vi "trace_math_spectra_divide.vi"(0 "reference in":refnum<class "OSA.lvclass">, 1 "spectrum 1 dividend trace idx":u32, 2 "spectrum 2 divisor trace idx":u32, 5 "error in (no error)":errorcluster) -> (13 "global dividend trace idx":u32, 14 "reference out":refnum<class "OSA.lvclass">, 19 "error out":errorcluster)   [LabVIEW 2010, in "OSA.lvclass"]
doc: "This divides two spectra On return will spectrum1 be equal to spectrum1 / spectrum2 \n\nParameters\n\nspectrum1: the dividend and also the output spectrum. \n\nspectrum2: the divisor. \n\nReturns FTS_ERROR_DIMENSION_MISMATCH if the lengths of the two spectra are different FTS_ERROR_DIMENSION_MISMATCH if the x-axis values of the two spectra differ FTS_SUCCESS on success"
uses:
  OSA.lvclass
  typeDef/acq_dataType.ctl
  FTSLib.dll
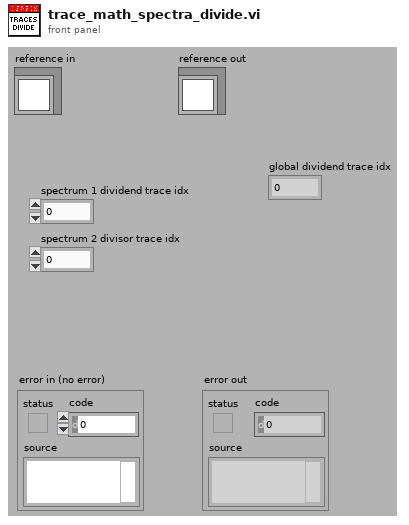
[diagram p1: front panel]
types:
  T1 = typedef "OSA.lvclass/acq_dataType.ctl" = enum16{"none", "interferogram", "spectrum"}
  T2 = typedef "OSA.lvclass/ObjectAttributes.ctl" = cluster{"Stop":bool, "dataType":T1, "spectrometerIdx":u16, "buffer size interferogram":i32, "interferogram":cluster{"new":bool, "plot_x_ min":sgl, "plot_x_max":sgl, "plot_y_min":sgl, "plot_y_max":sgl, "Graph Intrfrgrm":T3, "timeStamp":u32, "signal (%)":dbl, "traces":cluster{"idx":u32, "broadBand":bool, "monoChromatic":bool, "peakToPeakSignal":dbl, "peakToPeakPos":dbl}[], "traces idx last":i32}, "spectrum":cluster{"new":bool, "plot_x_min":sgl, "plot_x_max":sgl, "plot_unit_x":T4, "plot_unit_y":T5, "plot_y_min":sgl, "plot_y_max":sgl, "Graph Spectrum":T3, "timeStamp":u32, "X_VAL_OPTIONS":enum16{"MIN_MAX", "ARRAY"}, "traces":cluster{"idx":u32}[], "traces idx last":i32}, "Thorlabs_OSA_64.lvclass:queue_action.ctlqueue ref":refnum<queue>, "action":T6, "plot zoom step":dbl, "buffer semaphore":T7, "acq stopped":bool, "dataType active":T1, "temperature (degr C)":sgl, "pressure (hPa)":sgl, "rel humidity (%)":sgl, "settings":cluster{"resolution":u16, "sensitivity":u16, "Average":bool, "average nr":u32, "apodisation":T8, "acq delay (ms)":u32, "airMesure":T9, "wmtr on":bool, "intfgrm_smooth_width":u16, "intfgrm_smooth_nrOfPasses":u16, "intfgrm_smooth":T10, "phaseCorrection":T11, "zeroFill":u8, "spectr_smooth":T10, "spectr_smooth_width":u16, "spectr_smooth_nrOfPasses":u16, "resolution (/cm)":sgl, "REF wavelength, (nm)":dbl, "gain_idx":u16, "gainAuto":bool, "gain_relative":dbl, "PD sensitivity mode":T12, "PD senseMode implemented":bool, "SensorTemperature implemented":bool, "SensorPressure implemented":bool, "SensorHumidity implemented":bool, "attenuationAuto":bool, "attenuationOnOff":bool, "attenuationAvailable":bool, "offsetAvailable":bool, "offset":i32, "offset max":u16}, "peaks position":sgl[], "peaks width":sgl[], "peaks height":sgl[], "peaks max nr":u32, "peaks latest nr":i32, "peaks new":bool, "power":dbl, "power new":bool, "path":string, "wavelength (WNr)":dbl, "wavelength new":bool, "buffer size spectrum":i32, "status":string, "VI reference":refnum<vi>, "funcPointer":u64, "libraryPointer":u64, "singleAcquisition":bool, "coherenceLength (cm)":dbl, "coherenceLength new":bool, "spectrometer model":string, "spectrometer serial nr":string, "peaks thld left":sgl[], "peaks thld right":sgl[], "coherenceLength error (cm)":dbl, "ADC bits":u16, "peaks position centroid":sgl[], "peaks height centroid":sgl[], "OSA series":T13, "channel index spectrum":u16, "spectrometer rangeLow, (/cm)":dbl, "spectrometer rangeHigh, (/cm)":dbl, "channel index interferogram":u16}
  T3 = typedef "OSA.lvclass/graph_intensity.ctl" = refnum<vi>
  T4 = typedef "OSA.lvclass/spectrum_x_unit.ctl" = enum16{"wavenr/cm", "THz", "eV", "nm_air", "nm_vac"}
  T5 = typedef "OSA.lvclass/y_unit.ctl" = enum16{"ADC counts", "dBm pwr absolute", "dBm pwr density", "mW pwr absolute", "mW pwr density"}
  T6 = typedef "OSA.lvclass/queue_action.ctl" = enum16{"none", "stop", "GUI_plotInterferogram", "GUI_plotSpectrum", "GUI_plotInterferogramRescale", "GUI_plotSpectrumRescale", "GUI_plotInterferogramReset", "GUI_plotSpectrumReset", "GUI_plotInterferogramAutoScaleY", "GUI_plotSpectrumAutoScaleY", "GUI_plotInterferogramZoomOut", "GUI_plotSpectrumZoomOut", "GUI_plotInterferogramPane", "GUI_plotSpectrumPane", "GUI_plotInterferogramZoomMouse", "GUI_plotSpectrumZoomMouse", "GUI_spectrumChannelType", "GUI_channel", "ENVIRONMENT temperature", "ENVIRONMENT pressure", "MODE_resolution set", "MODE_resolution get", "MODE_sensitivity set", "MODE_sensitivity get", "MODE_PDTemperature set", "MODE_PDTemperature get", "REBOOT/RESET firmware", "ACQASYNC_acquireSingleSpectrum", "ACQASYNC_continuous start", "ACQASYNC_continuous stop\n", "ACQASYNC_get last interferogram", "ACQASYNC_get last spectrum", "ACQASYNC_get last waveNr", "ACQOPT_interferogram smoothing set", "ACQOPT_interferogram smoothing get", "ACQOPT_spectrum smoothing set", "ACQOPT_spectrum smoothing get", "ACQOPT_apodisation type set", "ACQOPT_apodisation type get", "ACQOPT_phase correction type set", "ACQOPT_phase correction type get", "ACQOPT_acqIntervall_set", "ACQOPT_acqIntervall_get", "ACQOPT_average spectrum set", "ACQOPT_average spectrum get", "ACQOPT_rolling average set", "ACQOPT_rolling average get", "ACQOPT_zero fill factor set", "ACQOPT_zero fill factor get", "ACQOPT_cycle counting set", "ACQOPT_cycle counting get", "ACQOPT_air measure option set", "ACQOPT_air measure option get", "ACQOPT_gainLevel auto get", "ACQOPT_gainLevel auto set", "ACQOPT_gainLevel get", "ACQOPT_gainLevel set", "ACQOPT_getAll", "INSTRUMENT_PROPERTY_range_WaveNr_min", "INSTRUMENT_PROPERTY_range_WaveNr_max", "INSTRUMENT_PROPERTY_reference_wavelength_cm^-1", "INSTRUMENT_PROPERTY_samplesPerRefPeriod", "INSTRUMENT_PROPERTY_resolution_waveNrPercm", "INSTRUMENT_PROPERTY_availableGainLevels", "INSTRUMENT_PROPERTY_status", "CONVERT", "ANALYSE_POWER", "ANALYSE_PEAKS", "ANALYSE_WAVELENGTH", "ANALYSE_SPECTRUM", "ANALYSE_INTERFEROGRAM", "ANALYSE_COHERENCE_LENGTH", "MATH", "MATH_power", "MATH_peaks", "FILE", "miscellaneous"}
  T7 = typedef "Semaphore RefNum" = refnum<k1>
  T8 = typedef "OSA.lvclass/apodisation.ctl" = enum16{"NONE", "NORTON_BEER_WEAK", "NORTON_BEER_MEDIUM", "NORTON_BEER_STRONG", "TRIANGULAR", "COSINE", "HANN", "HAMMING", "BLACKMANHARRIS3", "BLACKMANHARRIS4", "GAUSSIAN"}
  T9 = typedef "OSA.lvclass/airMeasure.ctl" = enum16{"TEMPERATURE", "PRESSURE"}
  T10 = typedef "OSA20X_misc.lvlib/interferogram_smoothing.ctl" = enum16{"NONE", "BINOMIAL", "SAVITSKY_GOLAY", "FOURIER", "MOVING_AVERAGE", "GAUSSIAN"}
  T11 = typedef "OSA.lvclass/phaseCorrection.ctl" = enum16{"NONE", "MERTZ", "FORMAN", "MERTZ_FILE", "FORMAN_FILE", "FUTURE COMP."}
  T12 = typedef "OSA20X_misc.lvlib/PDTemperatureMode.ctl" = enum16{"cool: better sensitivity/noise floor", "warm: extended wl range"}
  T13 = typedef "OSA.lvclass/OSA_series.ctl" = enum16{"OSA200", "OSA300", "UNKNOWN"}
  T14 = cluster{"idx":u32, "broadBand":bool, "monoChromatic":bool, "peakToPeakSignal":dbl, "peakToPeakPos":dbl}[]
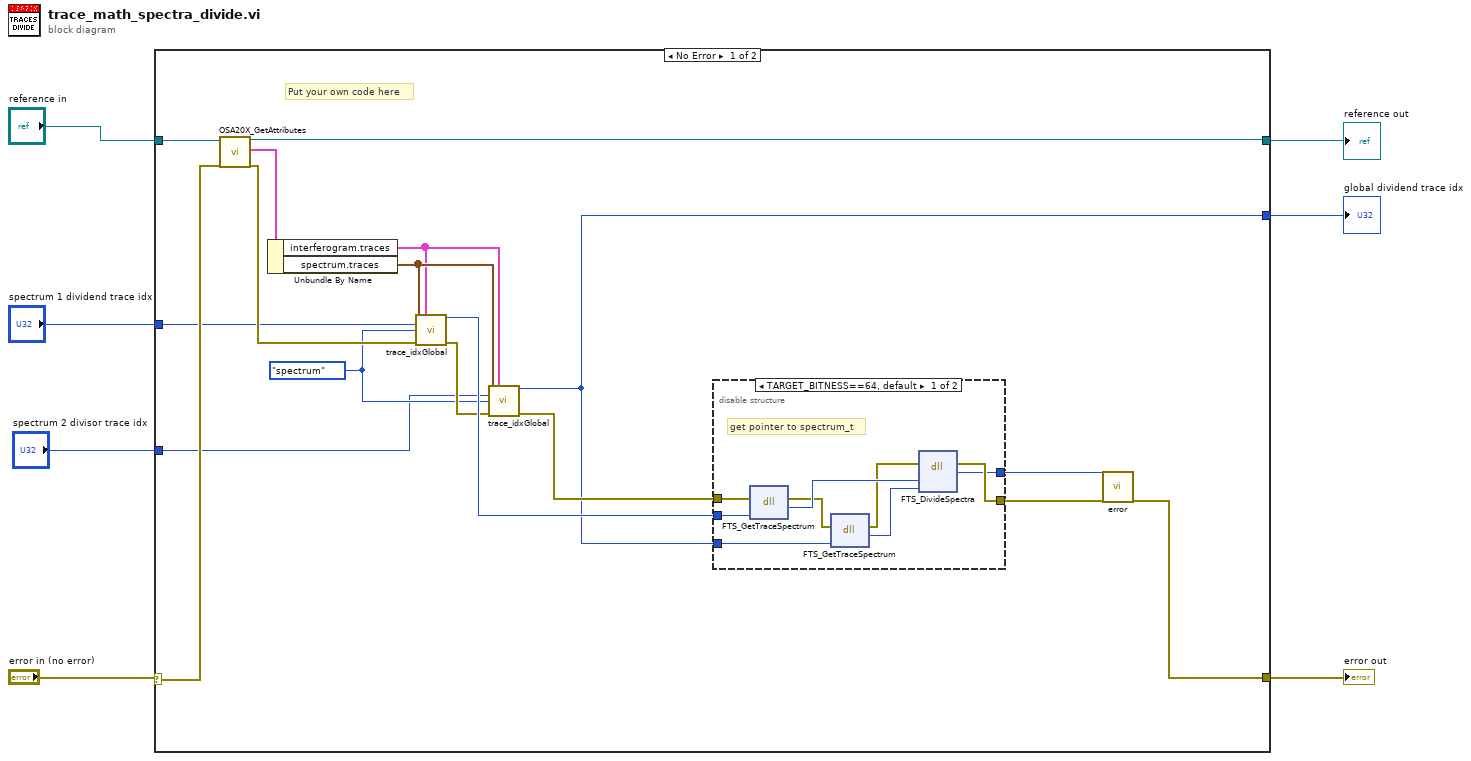
[diagram p0: block diagram]
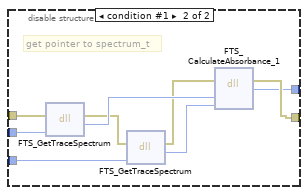
[diagram p2: hidden frame]
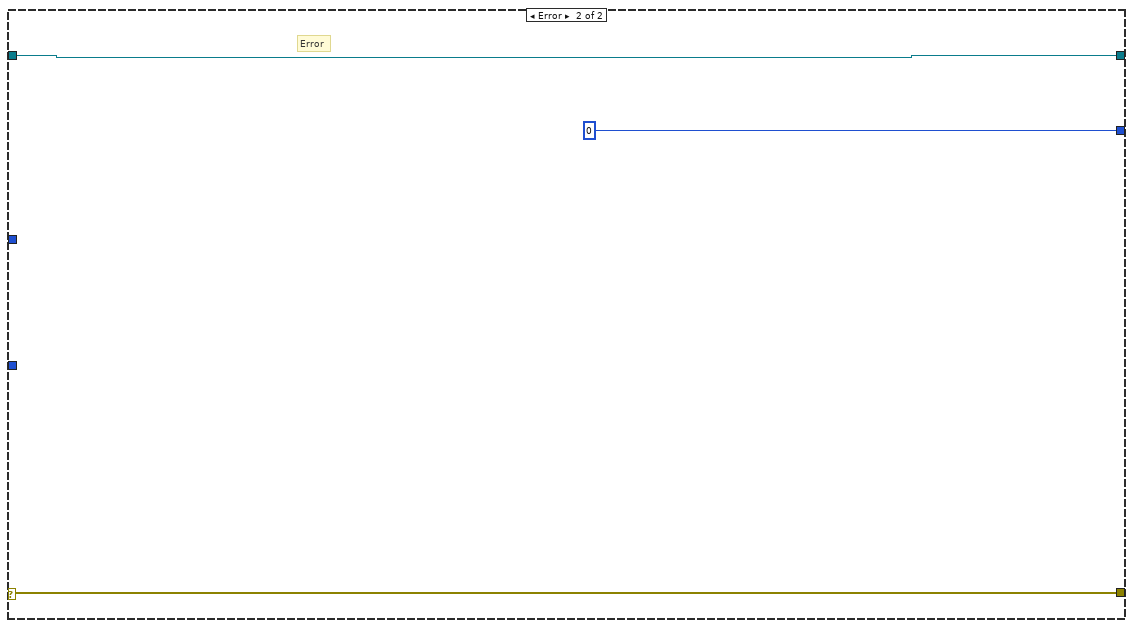
[diagram p3: hidden frame]
diagram:
  n1 = case shown="No Error" "error in (no error)" {
    selector: "error in (no error)" -> [w20 w45]
    tunnel: [w24 w45] -> w7
    tunnel: "reference in" -> [w22 w44]
    tunnel: [w21 w44] -> w2
    tunnel: "spectrum 1 dividend trace idx" -> [w18 _]
    tunnel: [w8 u32 0 ("global trace idx")] -> w3
    tunnel: "spectrum 2 divisor trace idx" -> [w9 _]
    frame No Error {
      w10 = acq_dataType."spectrum" ("dataType")
      # "Put your own code here"
      n2 = call "OSA20X_GetAttributes.vi"("reference in"=w22, "error in (no error)"=w20) -> ("reference out"=w21:refnum<class "OSA.lvclass">, "Data"=w23:T2, "error out"=w19:errorcluster)  [unwired: 14 in, 1 out]
      n3 = Unbundle By Name(w23) -> ("interferogram.traces"=w11:T14, "spectrum.traces"=w12:cluster{"idx":u32}[])
      n4 = call "trace_idxGlobal.vi"("traces_spectrum"=w12, "traces_interferogram"=w11, "trace idx"=w18, "dataType"=w10, "error in (no error)"=w19) -> ("global trace idx"=w15:u32, "error out"=w14:errorcluster)  [unwired: 9 in]
      n5 = call "trace_idxGlobal.vi"("traces_spectrum"=w12, "traces_interferogram"=w11, "trace idx"=w9, "dataType"=w10, "error in (no error)"=w14) -> ("global trace idx"=w8:u32, "error out"=w13:errorcluster)  [unwired: 9 in]
      n6 = disable-structure shown="TARGET_BITNESS==64, default" {
        disable-tunnel: w15 -> [w33 w35]
        disable-tunnel: w13 -> [w31 w36]
        disable-tunnel: [w30 w38] -> w17
        disable-tunnel: [w29 w37] -> w16
        disable-tunnel: w8 -> [w26 w34]
        frame condition #0 (active) {
          # "get pointer to spectrum_t"
          n7 = dll-call lib="FTSLib.dll" fn="FTS_GetTraceSpectrum"(error in=w31, "traceIdx"=w33) -> (error out=w28:errorcluster, "spectrum_t_pointer"=w32:u64)  [unwired: 3 in, 1 out]
          n8 = dll-call lib="FTSLib.dll" fn="FTS_GetTraceSpectrum"(error in=w28, "traceIdx"=w26) -> (error out=w27:errorcluster, "spectrum_t_pointer"=w25:u64)  [unwired: 3 in, 1 out]
          n9 = dll-call lib="FTSLib.dll" fn="FTS_DivideSpectra"(error in=w27, "spectrum_t_pointer"=w32, "spectrum_t_pointer"=w25) -> (error out=w30:errorcluster, "returnVal"=w29:i32)  [unwired: 4 in, 1 out]
        }
        frame condition #1 {
          # "get pointer to spectrum_t"
          n10 = dll-call lib="FTSLib.dll" fn="FTS_GetTraceSpectrum"(error in=w36, "traceIdx"=w35) -> (error out=w41:errorcluster, "spectrum_t_pointer"=w42:u32)  [unwired: 3 in, 1 out]
          n11 = dll-call lib="FTSLib.dll" fn="FTS_GetTraceSpectrum"(error in=w41, "traceIdx"=w34) -> (error out=w40:errorcluster, "spectrum_t_pointer"=w39:u32)  [unwired: 3 in, 1 out]
          n12 = dll-call lib="FTSLib.dll" fn="FTS_CalculateAbsorbance_1"(error in=w40, "spectrum_t_pointer"=w42, "spectrum_t_pointer"=w39) -> (error out=w38:errorcluster, "returnVal"=w37:i32)  [unwired: 4 in, 1 out]
        }
      }
      n13 = call "error.vi"("result code"=w16, "error in (no error)"=w17) -> ("error out"=w24:errorcluster)  [unwired: 15 in, 2 out]
    }
    frame Error {
      # "Error"
    }
  }
  "error out" <- w7
  "reference out" <- w2
  "global dividend trace idx" <- w3
